vi "Add N Packages to Feed.vi"(4 "create new package destination folderpath if none exists (F)":bool, 6 "package destination folderpath":path, 7 "create new feed if none exists (F)":bool, 8 "error in":errorcluster, 9 "overwrite existing packages (T)":bool=TRUE, 10 "package source filepaths":path[](array[path]), 11 "feed folderpath in":path) -> (0 "error out":errorcluster, 2 "package destination filepaths":path[](array[path]), 3 "feed folderpath out":path)   [LabVIEW 2014, in "NIPM_API.lvlib"]
doc: "Adds a package to a feed\n\nINPUT(s)\n<B>Feed folderpath</B>: Specifies the folder containing the feed\n\n<B>Package source filepaths</B>: Specifies the source filepaths of the packages to be added to the feed\n\n<B>Create new feed if none exists</B>: If this input is set to TRUE, this VI will create a new feed if there are no existing feed files in the specified feed folderpath.\n\n<B>Overwrite existing packages</B>: If this input is set to TRUE, this VI will copy the source packages to the package destination folderpath and overwrite an existing packages in the package destination folder if necessary.\n\n<B>Package destination folderpath</B>: If this input is left empty, this VI will default to using the feed folderpath as the package destination folderpath.\n\n<B>Create new package destination folder if none exists</B>: If this input is set to TRUE, this VI will create the package destination folder if it does not already exist.\n\nOUTPUT(s)\n<B>Feed folderpath out</B>: Outputs the specified feed folderpath\n\n<B>Package destination filepaths</B>: Outputs the destination filepaths of the packages that were added to the feed"
uses:
  NIPM_API.lvlib
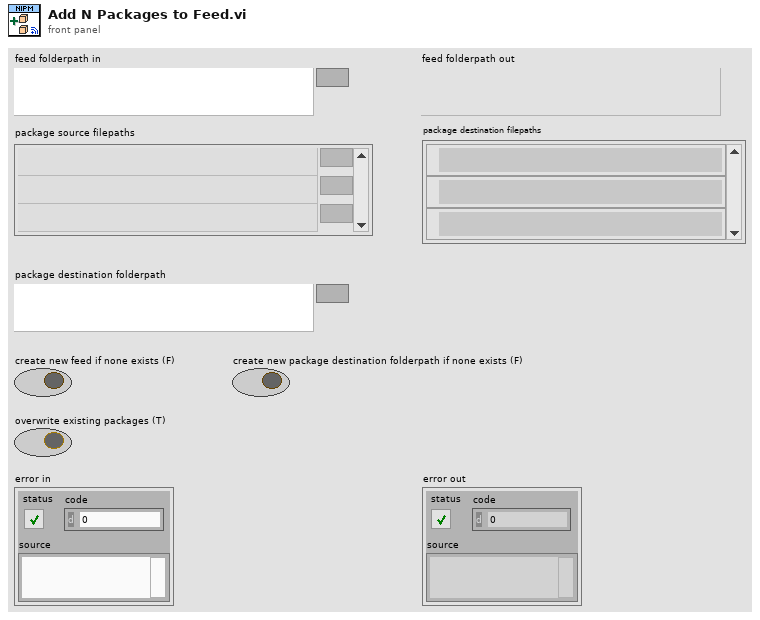
[diagram p1: front panel]
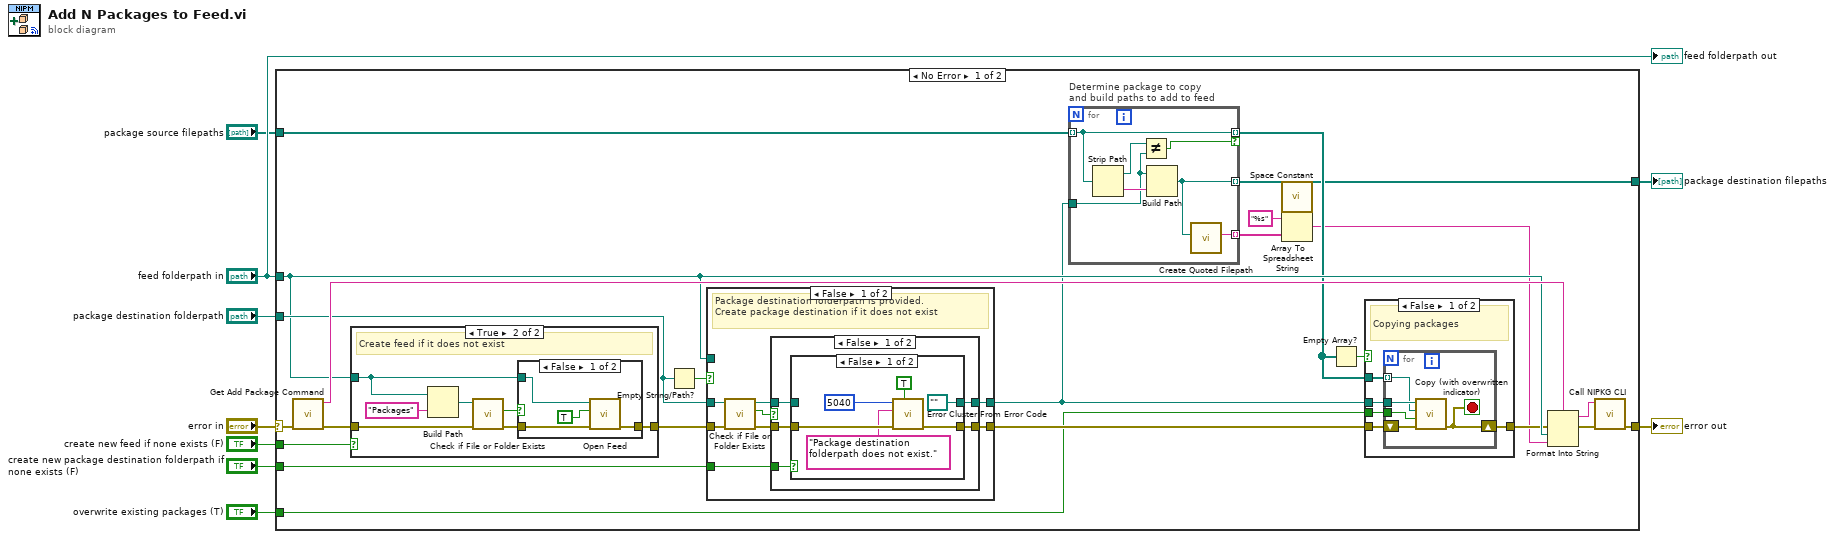
[diagram p0: block diagram]
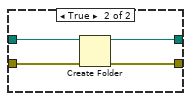
[diagram p3: hidden frame]
diagram:
  n1 = case shown="No Error" "error in" {
    selector: "error in" -> [w29 w92]
    tunnel: [w31 w92] -> w8
    tunnel: "feed folderpath in" -> [w22 _]
    tunnel: "create new feed if none exists (F)" -> [w27 _]
    tunnel: "package destination folderpath" -> [w25 _]
    tunnel: "create new package destination folderpath if none exists (F)" -> [w23 _]
    tunnel: "overwrite existing packages (T)" -> [w13 _]
    tunnel: "package source filepaths" -> [w21 _]
    tunnel: [w14 _] -> w1
    frame No Error {
      n2 = call "Get Add Package Command.vi"("error in (no error)"=w29) -> ("error out"=w28:errorcluster, "Add Package to Feed Command"=w30:string)  [unwired: 9 in]
      n3 = case shown="True" w27 {
        tunnel: w28 -> [w79 w84]
        tunnel: [w79 w81] -> w24
        tunnel: w22 -> [_ w80]
        frame False {
          # "Only use an existing feed"
        }
        frame True {
          # "Create feed if it does not exist"
          n4 = Build Path(base path=w80, name or relative path="Packages") -> (appended path=w85:path)
          n5 = call <vilib>:"Check if File or Folder Exists.vi"("error in (no error)"=w84, "path"=w85) -> ("error out"=w82:errorcluster, "file or folder exists?"=w83:bool)  [unwired: 7 in, 1 out]
          n6 = case shown="False" w83 {
            tunnel: w82 -> [w90 w91]
            tunnel: [w89 w91] -> w81
            tunnel: w80 -> [w88 _]
            frame False {
              n7 = call "Open Feed.vi"("error in"=w90, "create feed if necessary (F)"=TRUE, "feed folderpath"=w88) -> ("error out"=w89:errorcluster)  [unwired: 6 in, 2 out]
            }
            frame True {
            }
          }
        }
      }
      n8 = Empty String/Path?(string/path=w25) -> (empty?=w26:bool)
      n9 = case shown="False" w26 {
        tunnel: [w55 w77] -> w16
        tunnel: w25 -> [w59 _]
        tunnel: w23 -> [w54 _]
        tunnel: w24 -> [w58 w78]
        tunnel: [w52 w78] -> w17
        tunnel: w22 -> [_ w77]
        frame False {
          # "Package destination folderpath is provided.\nCreate package destination if it does not exist"
          n10 = call <vilib>:"Check if File or Folder Exists.vi"("error in (no error)"=w58, "path"=w59) -> ("error out"=w53:errorcluster, "file or folder exists?"=w57:bool, "dup path"=w56:path)  [unwired: 7 in]
          n11 = case shown="False" w57 {
            tunnel: w56 -> [w63 w76]
            tunnel: [w62 w76] -> w55
            tunnel: w54 -> [w64 _]
            tunnel: w53 -> [w61 w75]
            tunnel: [w60 w75] -> w52
            frame False {
              n12 = case shown="False" w64 {
                tunnel: w63 -> [_ w72]
                tunnel: [path "" ("dup path") w71] -> w62
                tunnel: w61 -> [w69 w74]
                tunnel: [w66 w73] -> w60
                frame False {
                  n13 = call <vilib>:"Error Cluster From Error Code.vi"("show call chain? (False)"=TRUE, "error in (no error)"=w69, "error message (\"\")"="Package destination folderpath does not exist.", "error code (0)"=5040) -> ("error out"=w66:errorcluster)  [unwired: 5 in]
                }
                frame True {
                  n14 = Create Folder(path (use dialog)=w72, error in=w74) -> (created path=w71:path, error out=w73:errorcluster)  [unwired: 1 in, 1 out]
                }
              }
            }
            frame True {
            }
          }
        }
        frame True {
          # "No destination specified\nStore packages in the feed's folder"
        }
      }
      n15 = for "Determine package to copy\nand build paths to add to feed" {
        tunnel: w21 -> [w50] mode=indexing
        tunnel: w16 -> [w48]
        tunnel: [w50] -> w15 mode=indexing if=w47
        tunnel: [w46] -> w19 mode=indexing
        tunnel: [w45] -> w14 mode=indexing
        n16 = Strip Path(path=w50) -> (stripped path=w49:path, name=w51:string)
        n17 = Not Equal?(x=w49, y=w48) -> (x != y?=w47:bool)
        n18 = Build Path(base path=w48, name or relative path=w51) -> (appended path=w45:path)
        n19 = call "Create Quoted Filepath.vi"("Path"=w45) -> ("Quoted Path String"=w46:string)  [unwired: 10 in]
      }
      n20 = call <vilib>:"Space Constant.vi"() -> ("String"=w20:string)
      n21 = Array To Spreadsheet String(delimiter (Tab)=w20, array=w19, 3:"%s" ("format string")) -> (spreadsheet string=w10:string)
      n22 = Empty Array?(array=w15) -> (empty?=w12:bool)
      n23 = case shown="False" w12 {
        tunnel: w17 -> [w38 w44]
        tunnel: w16 -> [w37 _]
        tunnel: w15 -> [w36 _]
        tunnel: w13 -> [w35 _]
        tunnel: [w34 w44] -> w11
        frame False {
          # "Copying packages"
          n24 = for {
            shift-right: [w39] -> w34
            shift-left: w38 -> [w43]
            tunnel: w37 -> [w42]
            tunnel: w36 -> [w41] mode=indexing
            tunnel: w35 -> [w40]
            stop <- w39 stop-if-true
            n25 = call "Copy (with overwritten indicator).vi"("error in (no error)"=w43, "overwrite (F)"=w40, "source filepath"=w41, "target folderpath"=w42) -> ("error out"=w39:errorcluster)  [unwired: 5 in, 2 out]
          }
        }
        frame True {
          # "No packages needing to be copied"
        }
      }
      n26 = Format Into String(format string=w30, error in=w11, w22, w10) -> (resulting string=w33:string, error out=w32:errorcluster)  [unwired: 1 in]
      n27 = call "Call NIPKG CLI.vi"("error in (no error)"=w32, "command"=w33) -> ("error out"=w31:errorcluster)  [unwired: 8 in, 1 out]
    }
    frame Error {
    }
  }
  "error out" <- w8
  "package destination filepaths" <- w1
  "feed folderpath out" <- "feed folderpath in"
